vi "Restartable Demo.vi"() -> ()   [LabVIEW 2022 SP3]
uses:
  Flex/Publish Element.vi
  Flex/Instantiate.vi
  Flex/))Channel.vi
  Flex/Check Room in Queues.vi
  Flex/Flex.lvlib
panel:
  in  "Release 3":bool
  in  "Start 3":bool
  in  "Release 2":bool
  in  "Start 2":bool
  in  "Release":bool
  in  "Start":bool
  in  "Slide":dbl(slide) scale=0.0..10.0
  in  "Stop":bool
  out "Rate":u32
  out "5mS":dbl(graph)
  out "20mS":dbl(graph)
  out "50mS":dbl(graph)
  out "Count":i32[](array[numeric])
  out "Buffers":dbl[](array[slide]) scale=0.0..1.0
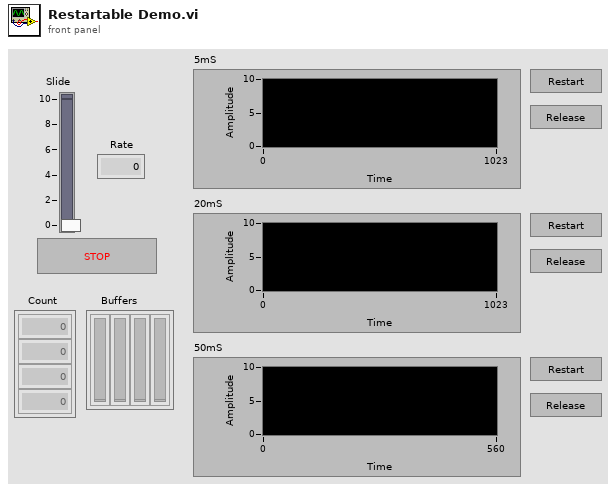
[diagram p1: front panel]
types:
  T1 = typedef "Flex.lvlib/))Channel.ctl" = refnum<queue>
  T2 = typedef "Flex.lvlib/Element.ctl" = dbl
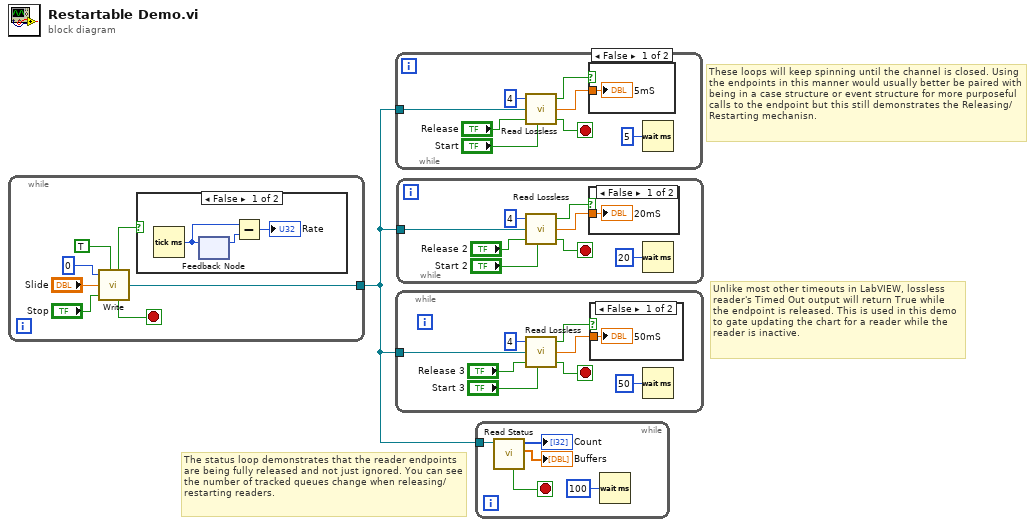
[diagram p0: block diagram]
diagram:
  # "The status loop demonstrates that the reader endpoints are being fully released and not just ignored. You can see the number of tracked queues change when releasing/restarting readers."
  # "Unlike most other timeouts in LabVIEW, lossless reader's Timed Out output will return True while the endpoint is released. This is used in this demo to gate updating the chart for a reader while the reader is inactive."
  # "These loops will keep spinning until the channel is closed. Using the endpoints in this manner would usually better be paired with being in a case structure or event structure for more purposeful calls to the endpoint but this still demonstrates the Releasing/Restarting mechanisn."
  n1 = while {
    tunnel: [w6] -> w1
    stop <- w5 stop-if-true
    n2 = call "Write.vi"("Timeout mS (-1)"=0, "Synchronous (F)"=TRUE, "element"="Slide", "Close? (F)"="Stop") -> ("Timed Out?"=w3:bool, "channel"=w6:T1, "Closed?"=w5:bool)  [unwired: 3 in]
    n3 = case shown="False" w3 {
      frame False {
        n4 = Tick Count (ms)() -> (millisecond timer value=w10:u32)
        n5 = feedback #1() -> (w9:u32)  [unwired: 1 in]
        n6 = feedback-in #1(w10) -> ()
        n7 = Subtract(x=w10, y=w9) -> (x-y=→"Rate":u32)
      }
      frame True {
      }
    }
  }
  n8 = while {
    tunnel: w1 -> [w19]
    stop <- w15 stop-if-true
    n9 = call "Read Lossless.vi"("Depth (Unlimited)"=4, "FlexChannel"=w19, "Release (F)"="Release", "Restart (F)"="Start") -> ("Timed Out?"=w12:bool, "Element"=w18:T2, "Closed?"=w15:bool)  [unwired: 3 in]
    n10 = case shown="False" w12 {
      tunnel: w18 -> [w20 _]
      frame False {
        "5mS" <- w20
      }
      frame True {
      }
    }
    n11 = Wait (ms)(milliseconds to wait=u32 5) -> ()  [unwired: 1 out]
  }
  n12 = while {
    tunnel: w1 -> [w28]
    stop <- w24 stop-if-true
    n13 = call "Read Lossless.vi"("Depth (Unlimited)"=4, "FlexChannel"=w28, "Release (F)"="Release 3", "Restart (F)"="Start 3") -> ("Timed Out?"=w21:bool, "Element"=w27:T2, "Closed?"=w24:bool)  [unwired: 3 in]
    n14 = case shown="False" w21 {
      tunnel: w27 -> [w29 _]
      frame False {
        "50mS" <- w29
      }
      frame True {
      }
    }
    n15 = Wait (ms)(milliseconds to wait=u32 50) -> ()  [unwired: 1 out]
  }
  n16 = while {
    tunnel: w1 -> [w37]
    stop <- w33 stop-if-true
    n17 = call "Read Lossless.vi"("Depth (Unlimited)"=4, "FlexChannel"=w37, "Release (F)"="Release 2", "Restart (F)"="Start 2") -> ("Timed Out?"=w30:bool, "Element"=w36:T2, "Closed?"=w33:bool)  [unwired: 3 in]
    n18 = case shown="False" w30 {
      tunnel: w36 -> [w38 _]
      frame False {
        "20mS" <- w38
      }
      frame True {
      }
    }
    n19 = Wait (ms)(milliseconds to wait=u32 20) -> ()  [unwired: 1 out]
  }
  n20 = while {
    tunnel: w1 -> [w42]
    stop <- w41 stop-if-true
    n21 = call "Read Status.vi"("channel"=w42) -> ("Usage Ratio"=→"Buffers":dbl[], "Queued Count"=→"Count":i32[], "Closed?"=w41:bool)  [unwired: 4 in, 4 out]
    n22 = Wait (ms)(milliseconds to wait=u32 100) -> ()  [unwired: 1 out]
  }
